vi "Update.vi"(8 "error in (no error)":errorcluster, 10 "Message in":refnum<class "UpdateMessage.lvclass">, 11 "Piezo in":refnum<class "Piezo.lvclass">) -> (0 "error out":errorcluster, 3 "Piezo out":refnum<class "Piezo.lvclass">)   [LabVIEW 2012, in "Piezo.lvclass"]
doc: "The update method processes the command 'update'. \n\nThe command 'update' is used for receiving new values to be set to the private data of the class. This could be seen as a public set method for setting new parameters to the private class data."
uses:
  Piezo.lvclass
  <vilib>/Distrio/Murmex/UpdateMessage/UpdateMessage.lvclass
  Piezo.lvclass/Piezo.ctl
  <vilib>/Distrio/Murmex/Murmex/Murmex.lvclass
panel:
  # "This method is called when the UPDATE\ntrigger is sent. \n\nOverride this method when your component needs to\nrespond to this trigger. \n\nCall parent for proper implementation"
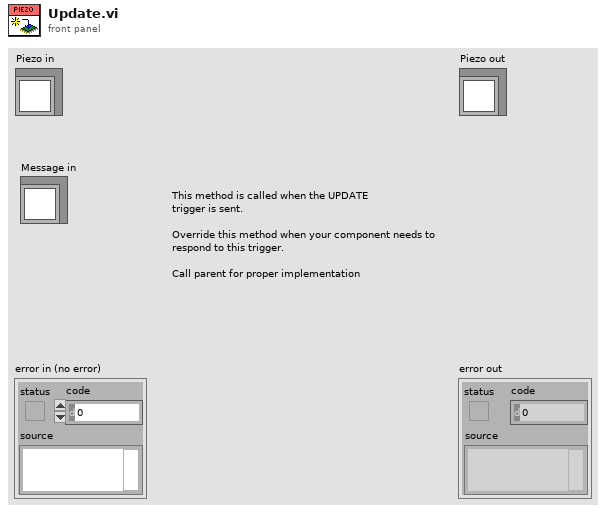
[diagram p1: front panel]
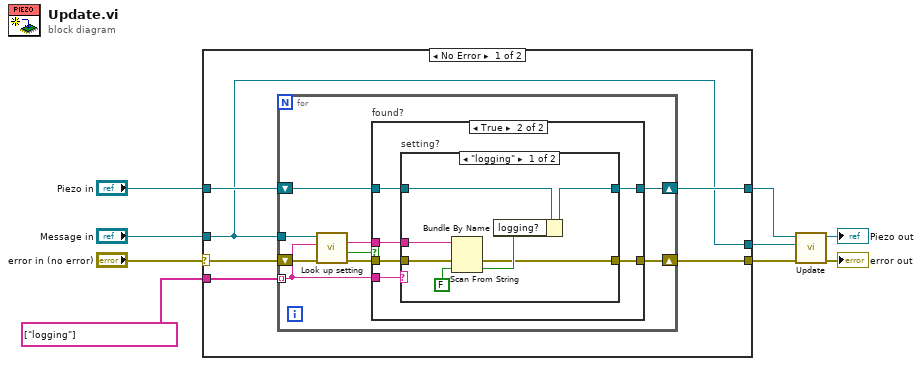
[diagram p0: block diagram]
diagram:
  n1 = case shown="No Error" "error in (no error)" {
    selector: "error in (no error)" -> [w14 w44]
    tunnel: [w11 w44] -> w6
    tunnel: [w12 w43] -> w5
    tunnel: "Piezo in" -> [w13 w43]
    tunnel: [w10 w42] -> w3
    tunnel: "Message in" -> [w10 w42]
    tunnel: string[] ["logging"] ("key chains") -> [w15 _]
    frame No Error {
      n2 = for {
        tunnel: w15 -> [w20] mode=indexing
        tunnel: w10 -> [w24]
        shift-right: [w18] -> w11
        shift-left: w14 -> [w23]
        shift-right: [w17] -> w12
        shift-left: w13 -> [w19]
        n3 = call <vilib>:"Look up setting.vi"("error in (no error)"=w23, "tag name"=w20, "UpdateMessage in"=w24) -> ("error out"=w21:errorcluster, "found?"=w22:bool, "value"=w16:string)  [unwired: 5 in, 1 out]
        n4 = case "found?" shown="True" w22 {
          tunnel: w21 -> [w25 w29]
          tunnel: w20 -> [_ w32]
          tunnel: w19 -> [w26 w31]
          tunnel: [w25 w30] -> w18
          tunnel: [w26 w28] -> w17
          tunnel: w16 -> [_ w27]
          frame False {
          }
          frame True {
            n5 = case "setting?" shown="\"logging\"" w32 {
              tunnel: w31 -> [w39 w40]
              tunnel: [w33 w41] -> w30
              tunnel: w29 -> [w37 w41]
              tunnel: [w38 w40] -> w28
              tunnel: w27 -> [w36 _]
              frame "logging" {
                n6 = Scan From String(input string=w36, error in=w37, default 1=FALSE ("settings.logging?")) -> (error out=w33:errorcluster, output 1=w34:bool)  [unwired: 2 in, 2 out]
                n7 = Bundle By Name(cluster=w39, "logging?"=w34) -> (w38:refnum<class "Piezo.lvclass">)
              }
              frame Default {
              }
            }
          }
        }
      }
    }
    frame Error {
    }
  }
  n8 = call-parent "Update.vi"("error in (no error)"=w6, "Message in"=w3, "Murmex in"=w5) -> ("error out"=→"error out":errorcluster, "Murmex out"=→"Piezo out":refnum<class "Piezo.lvclass">)  [unwired: 7 in]
